vi "Main.vi"() -> ()   [LabVIEW 2020]
doc: "This template is for the Queued Message Handler design pattern.\n\nThe Event Handling Loop generates messages based on user interface actions.\n\nThe Message Handling Loop processes messages generated by the Event Handling Loop, or by other messages. The messages are string values, so new messages can be added easily to the Message Cases case structure in the Message Handling Loop. Each message cluster can also provide an optional value for Message Data, which is a variant that can be converted to whatever message-specific data is required."
uses:
  <vilib>/numeric/Random Number (Range) I64.vi
  <vilib>/numeric/sub_Random U32.vi
  <vilib>/Utility/error.llb/Error Cluster From Error Code.vi
  <vilib>/ErrorRing/Error Ring.xnode
  support/Message Queue/Message Queue.lvlib
  support/User Event - Stop/User Event - Stop.lvlib
panel:
  out "Order Array Display":string[](array[string])
  out "Button Array":refnum<vi>[](array[refnum])
  out "Stage Num":i32
  out "Click Num":i32
  out "Display <Replace Me>":string
  in  "Blue":bool
  in  "Red":bool
  in  "Exit":bool
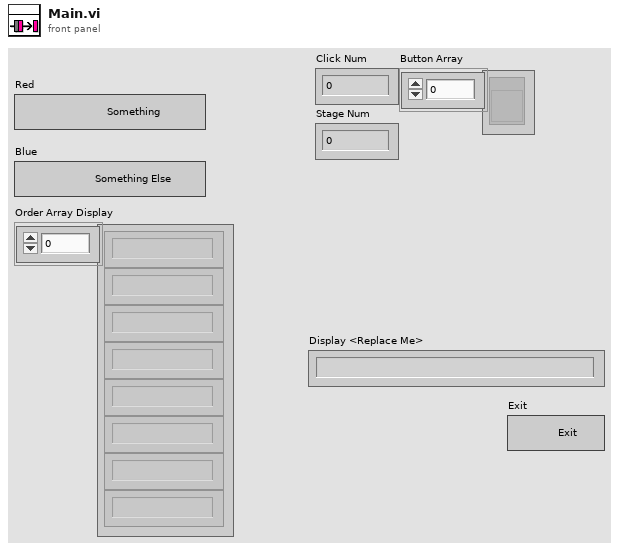
[diagram p1: front panel]
types:
  T1 = typedef "Message Queue.lvlib/All Message Queues.ctl" = cluster{"UI":refnum<queue>}
  T2 = enum8{"Enabled", "Disabled", "Disabled and Grayed Out"}
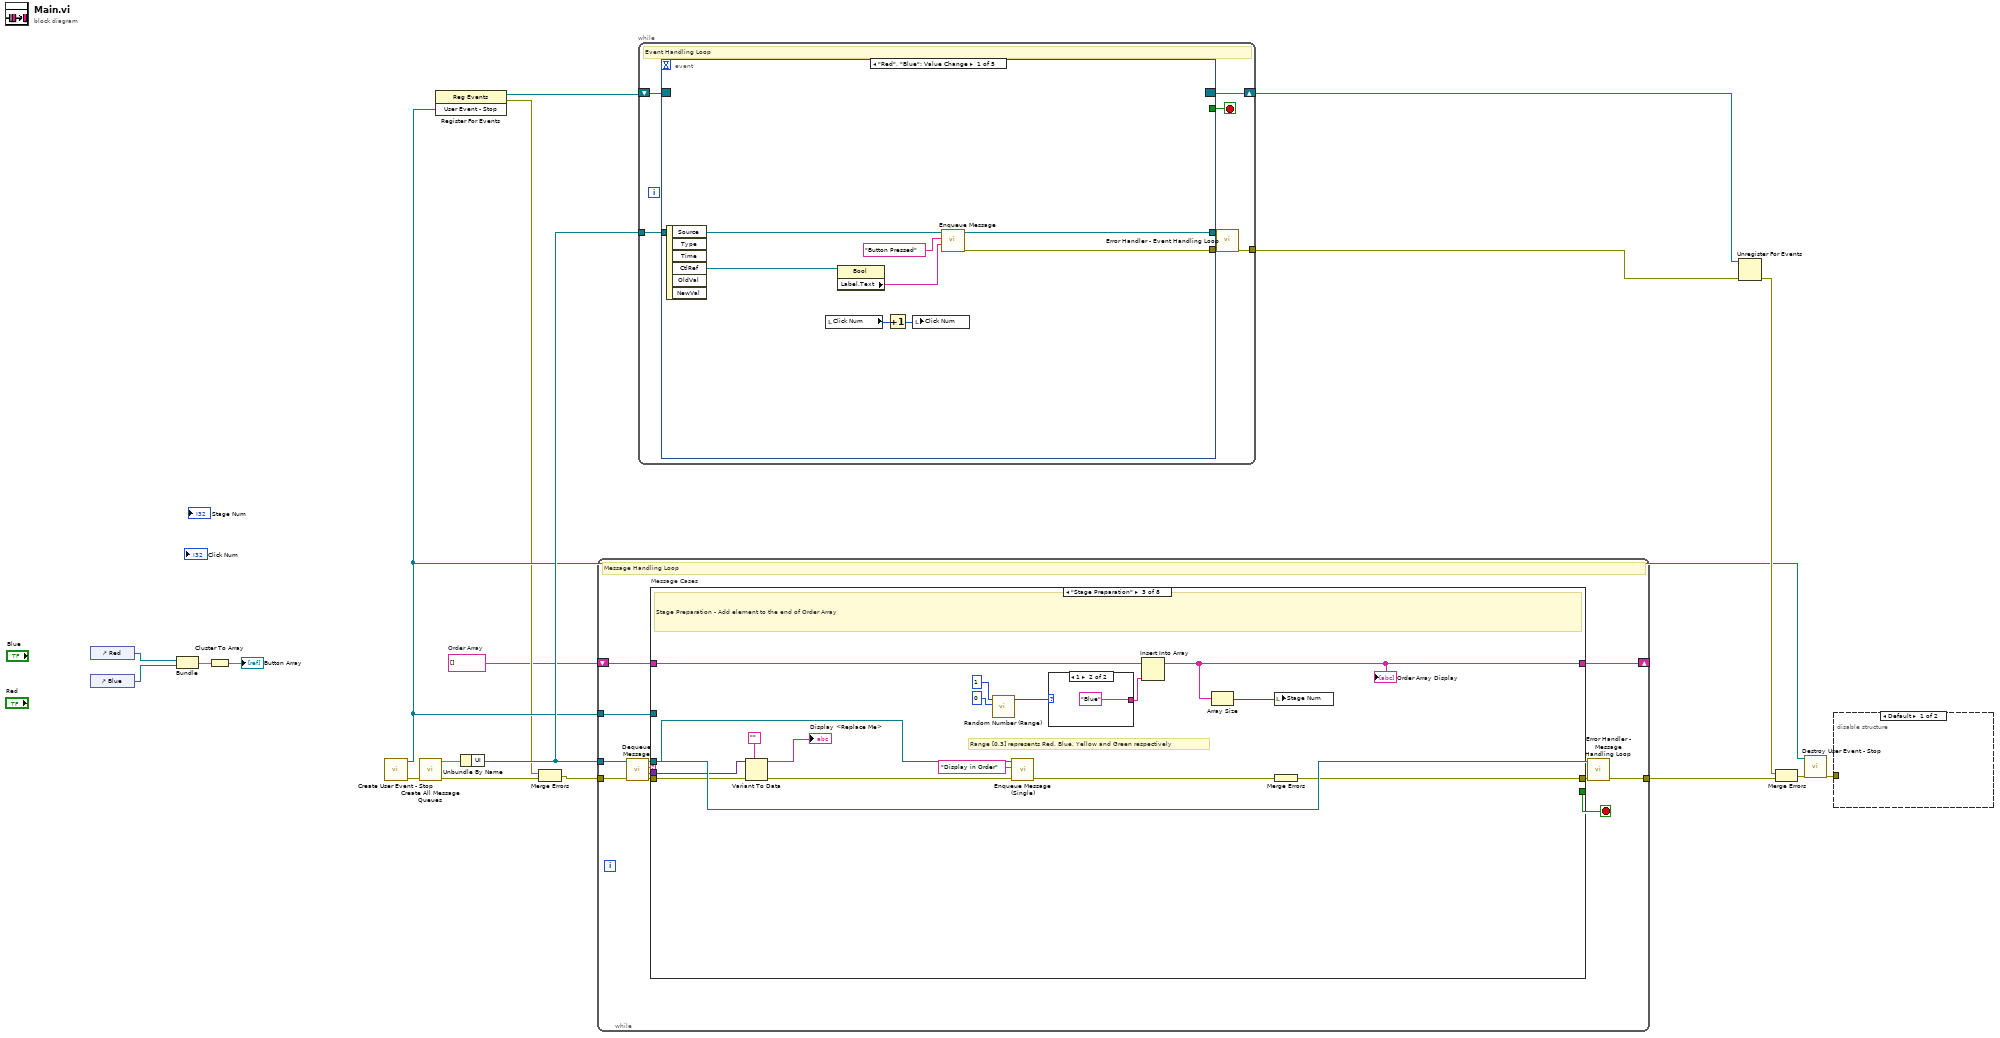
[diagram p0: block diagram]
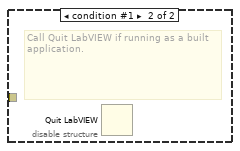
[diagram p2: hidden frame]
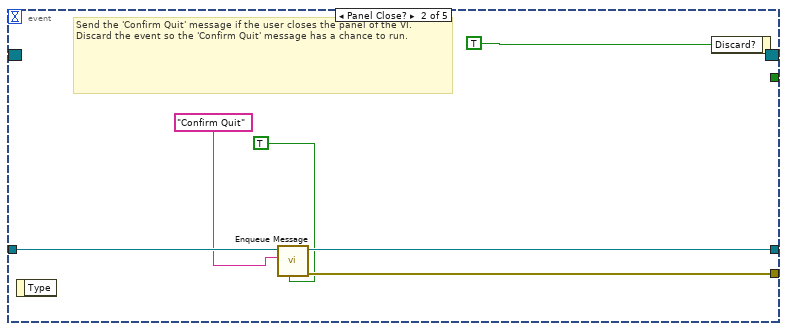
[diagram p3: hidden frame]
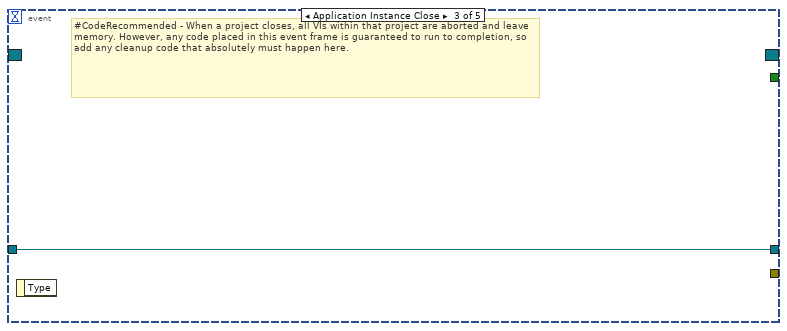
[diagram p4: hidden frame]
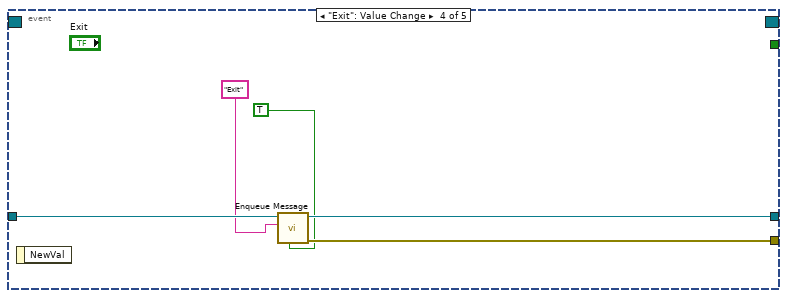
[diagram p5: hidden frame]
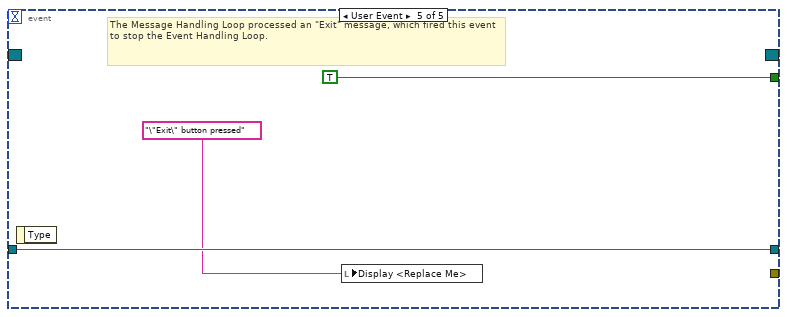
[diagram p6: hidden frame]
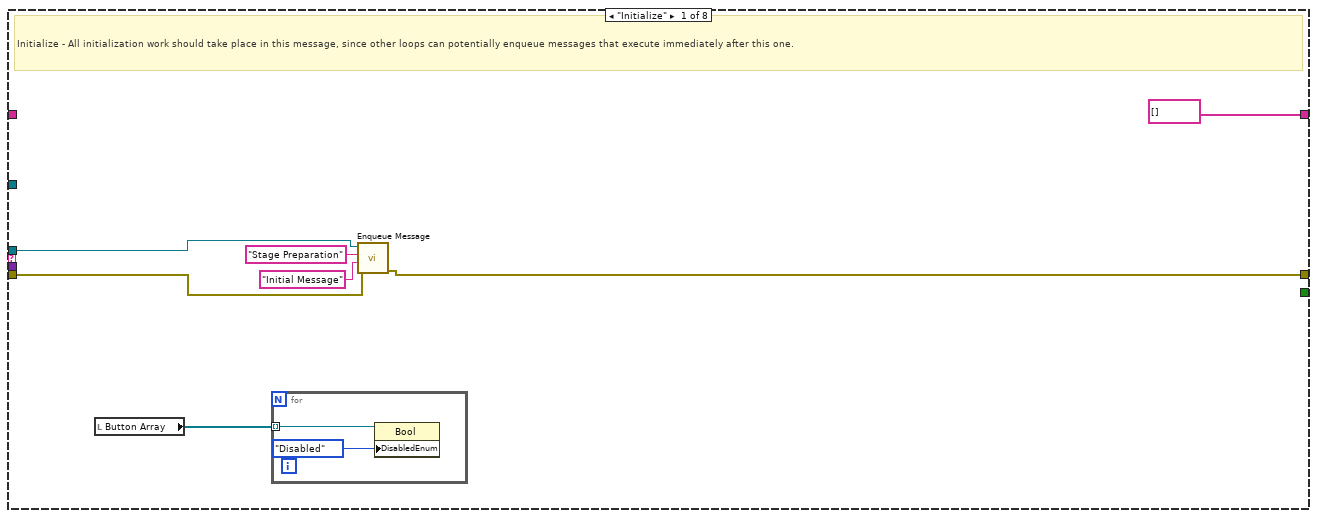
[diagram p7: hidden frame]
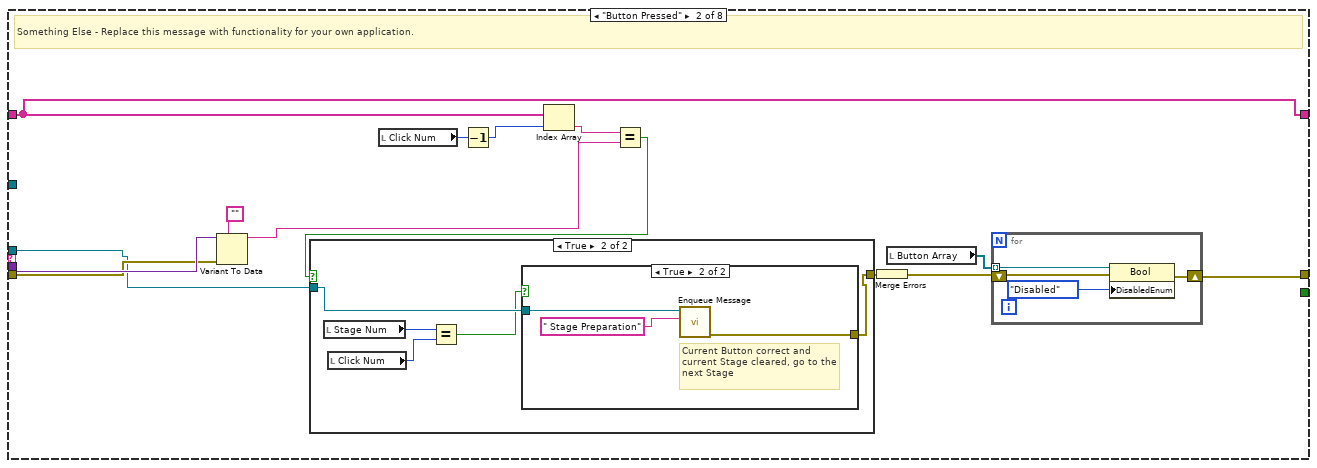
[diagram p8: hidden frame]
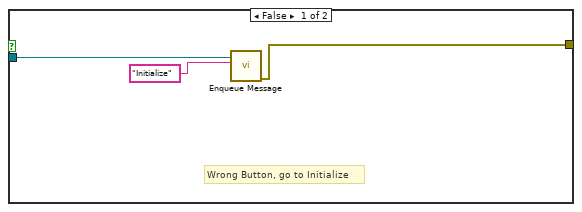
[diagram p9: hidden frame]
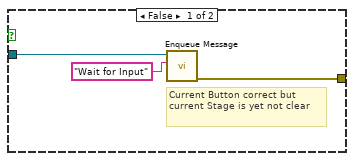
[diagram p10: hidden frame]
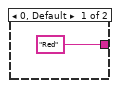
[diagram p11: hidden frame]
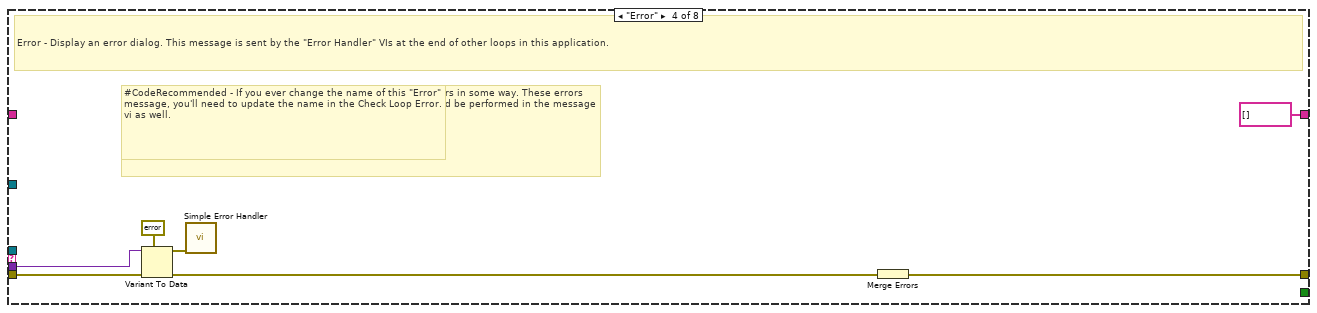
[diagram p12: hidden frame]
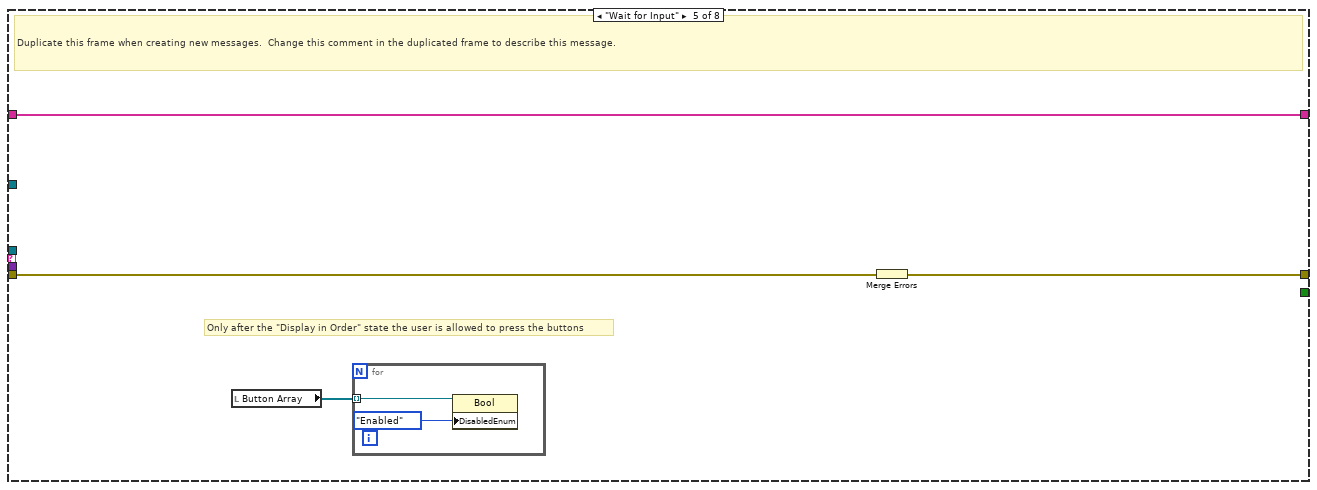
[diagram p13: hidden frame]
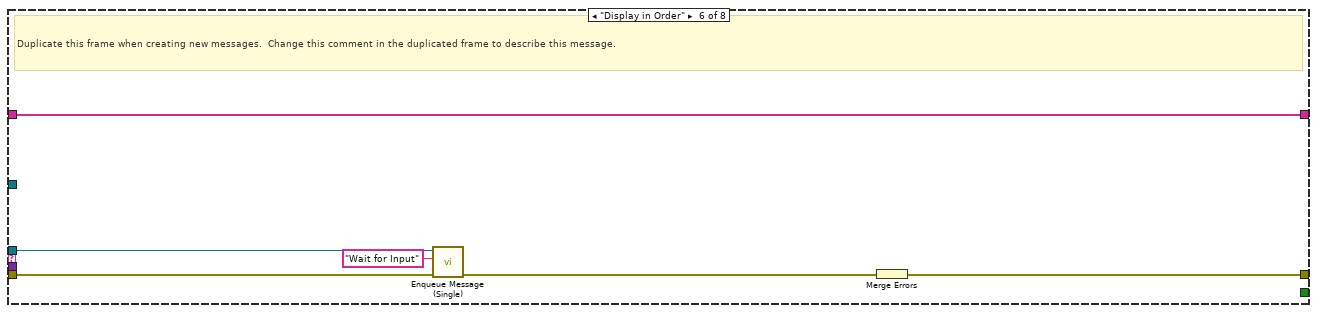
[diagram p14: hidden frame]
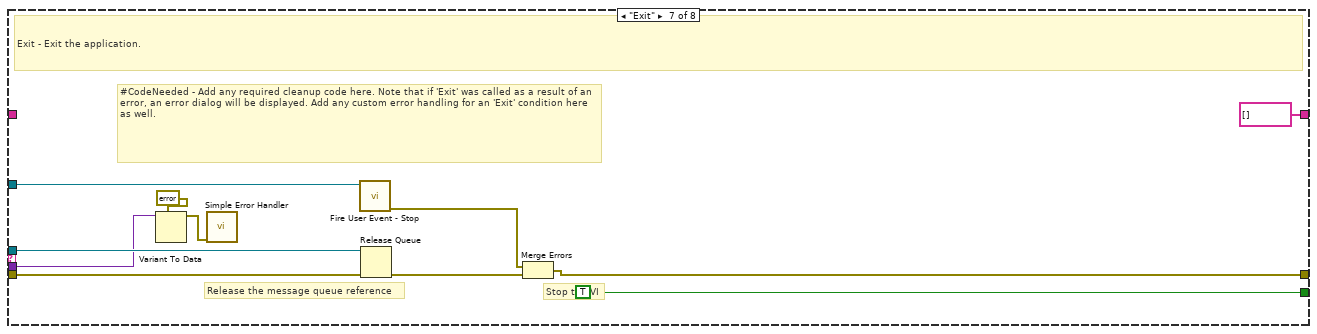
[diagram p15: hidden frame]
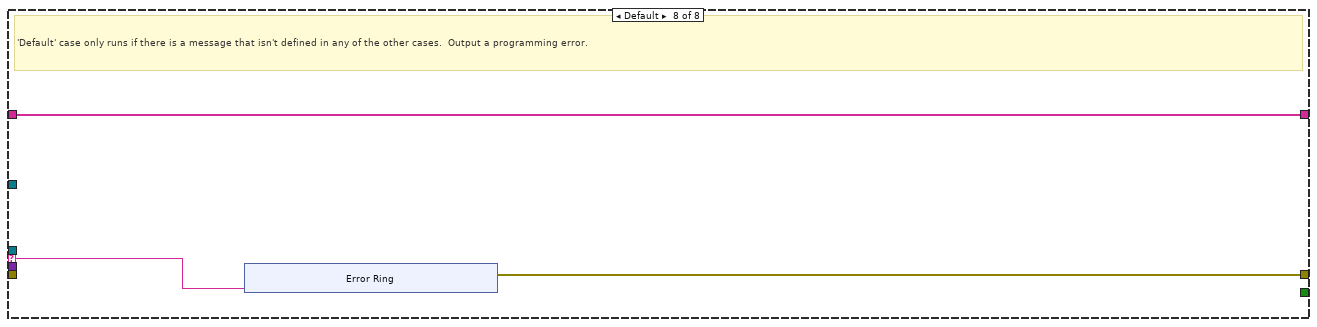
[diagram p16: hidden frame]
diagram:
  w5 = string[] []  # Order Array
  n1 = control-ref of="Red"() -> (w4:refnum<vi>)
  n2 = control-ref of="Blue"() -> (w3:refnum<vi>)
  n3 = Bundle("Red"=w4, "Blue"=w3) -> (w2:cluster{"Red":refnum<vi>, "Blue":refnum<vi>})  [unwired: 1 in]
  n4 = Cluster To Array(cluster=w2) -> (array=→"Button Array":refnum<vi>[])
  n5 = call "Create User Event - Stop.vi"() -> ("error out"=w15:errorcluster, "User Event - Stop"=w8:refnum<user-event>)  [unwired: 10 in]
  n6 = call "Create All Message Queues.vi"("error in (no error)"=w15) -> ("error out"=w19:errorcluster, "Message Queues out"=w18:T1)  [unwired: 9 in]
  n7 = register-events(w8) -> (reference out=w9:refnum<event-registration>, error out=w6:errorcluster)  [unwired: 2 in]
  n8 = Unbundle By Name(w18) -> ("UI"=w16:refnum<queue>)
  n9 = Merge Errors(w6, w19) -> (w7:errorcluster)
  n10 = while {
    tunnel: w16 -> [w25]
    tunnel: w8 -> [w30]
    tunnel: w7 -> [w29]
    tunnel: [w23] -> w17
    shift-right: [w20] -> _
    shift-left: w5 -> [w21]
    stop <- w31 stop-if-true
    # "Message Handling Loop"
    n11 = call "Dequeue Message.vi"("error in (no error)"=w29, "Message Queue"=w25) -> ("error out"=w28:errorcluster, "Message Data"=w26:variant, "Message"=w27:string, "dup Message Queue"=w24:refnum<queue>)  [unwired: 6 in]
    n12 = case "Message Cases" shown="\"Stage Preparation\"" w27 {
      selector: w27 -> [_ _ _ _ _ _ _ w122]
      tunnel: w24 -> [w35 w48 w74 _ _ w105 w120 _]
      tunnel: w28 -> [w37 w51 w87 w97 w101 w109 w114 _]
      tunnel: [w38 w42 w88 w92 w100 w108 w117 w123] -> w22
      tunnel: [_ _ _ _ _ _ TRUE _] -> w31
      tunnel: w26 -> [_ w52 w86 w96 _ _ w111 _]
      tunnel: w30 -> [_ _ _ _ _ _ w116 _]
      tunnel: w21 -> [_ w54 w82 _ w98 w107 _ w121]
      tunnel: [string[] [] w54 w77 string[] [] ("Order Array") w98 w107 string[] [] ("Order Array") w121] -> w20
      frame "Initialize" {
        # "Initialize - All initialization work should take place in this message, since other loops can potentially enqueue messages that execute immediately after this one."
        n13 = local read "Button Array"() -> (w33:refnum<vi>[])
        n14 = for {
          tunnel: w33 -> [w40] mode=indexing
          n15 = property class="Bool"(reference=w40, "DisabledEnum"=T2."Disabled" ("Disabled")) -> ()  [unwired: 1 in, 2 out]
        }
        n16 = call-poly "Enqueue Message.vi"("error in (no error)"=w37, "Message Data"="Initial Message" ("Initial Message"), "Message"="Stage Preparation", "Message Queue"=w35) -> ("error out"=w38:errorcluster)  [unwired: 6 in, 1 out]
      }
      frame "Button Pressed" {
        # "Something Else - Replace this message with functionality for your own application."
        n17 = Variant To Data(error in=w51, type="", Variant=w52) -> (data=w50:string)  [unwired: 1 out]
        n18 = local read "Click Num"() -> (w46:i32)
        n19 = Decrement(x=w46) -> (x-1=w45:i32)
        n20 = Index Array(array=w54, index=w45) -> (element=w44:string)
        n21 = Equal?(x=w44, y=w50) -> (x = y?=w49:bool)
        n22 = case shown="True" w49 {
          tunnel: w48 -> [w61 w65]
          tunnel: [w60 w66] -> w47
          frame False {
            # "Wrong Button, go to Initialize"
            n23 = call-poly "Enqueue Message.vi"("Message"="Initialize", "Message Queue"=w61) -> ("error out"=w60:errorcluster)  [unwired: 8 in, 1 out]
          }
          frame True {
            n24 = local read "Stage Num"() -> (w64:i32)
            n25 = local read "Click Num"() -> (w63:i32)
            n26 = Equal?(x=w64, y=w63) -> (x = y?=w62:bool)
            n27 = case shown="True" w62 {
              tunnel: [w69 w71] -> w66
              tunnel: w65 -> [w67 w72]
              frame False {
                # "Current Button correct but \ncurrent Stage is yet not clear"
                n28 = call-poly "Enqueue Message.vi"("Message"="Wait for Input", "Message Queue"=w67) -> ("error out"=w69:errorcluster)  [unwired: 8 in, 1 out]
              }
              frame True {
                # "Current Button correct and \ncurrent Stage cleared, go to the next Stage"
                n29 = call-poly "Enqueue Message.vi"("Message"=" Stage Preparation", "Message Queue"=w72) -> ("error out"=w71:errorcluster)  [unwired: 8 in, 1 out]
              }
            }
          }
        }
        n30 = Merge Errors(w47) -> (w43:errorcluster)
        n31 = local read "Button Array"() -> (w41:refnum<vi>[])
        n32 = for {
          tunnel: w41 -> [w58] mode=indexing
          shift-right: [w55] -> w42
          shift-left: w43 -> [w56]
          n33 = property class="Bool"(reference=w58, error in=w56, "DisabledEnum"=T2."Disabled" ("Disabled")) -> (error out=w55:errorcluster)  [unwired: 1 out]
        }
      }
      frame "Stage Preparation" {
        # "Range [0,3] represents Red, Blue, Yellow and Green respectively"
        # "Stage Preparation - Add element to the end of Order Array"
        n34 = Variant To Data(error in=w87, type="", Variant=w86) -> (data=→"Display <Replace Me>":string, error out=w84:errorcluster)
        n35 = call-poly <vilib>:"Random Number (Range).vi"("lower bound (-100)"=i64 0, "upper bound (100)"=i64 1) -> ("number"=w79:i64)  [unwired: 9 in]
        n36 = call "Enqueue Message (Single).vi"("error in (no error)"=w84, "Message"="Display in Order", "Message Queue"=w74) -> ("error out"=w75:errorcluster)  [unwired: 7 in, 1 out]
        n37 = case shown="1" w79 {
          tunnel: ["Red" "Blue"] -> w78
          frame 0, Default {
          }
          frame 1 {
          }
        }
        n38 = Insert Into Array(array=w82, new element=w78) -> (w77:string[])  [unwired: 1 in]
        "Order Array Display" <- w77
        n39 = Array Size(array=w77) -> (size(s)=w76:i32)
        n40 = local write "Stage Num"(w76) -> ()
        n41 = Merge Errors(w75) -> (w88:errorcluster)
      }
      frame "Error" {
        # "#CodeRecommended - If you ever change the name of this \"Error\" message, you'll need to update the name in the Check Loop Error.vi as well."
        # "#CodeRecommended - Consider creating a system for logging errors in some way. These errors are for notification purposes only. Handling of specific errors should be performed in the message frames that generated the error."
        # "Error - Display an error dialog. This message is sent by the \"Error Handler\" VIs at the end of other loops in this application."
        n42 = Variant To Data(error in=w97, type=errorcluster {"status"=FALSE, "code"=0, "source"=""} ("error constant"), Variant=w96) -> (data=w94:errorcluster, error out=w93:errorcluster)
        n43 = call <vilib>:"Simple Error Handler.vi"("error in (no error)"=w94) -> ()  [unwired: 4 in, 5 out]
        n44 = Merge Errors(w93) -> (w92:errorcluster)
      }
      frame "Wait for Input" {
        # "Only after the \"Display in Order\" state the user is allowed to press the buttons"
        # "Duplicate this frame when creating new messages.  Change this comment in the duplicated frame to describe this message."
        n45 = local read "Button Array"() -> (w99:refnum<vi>[])
        n46 = for {
          tunnel: w99 -> [w103] mode=indexing
          n47 = property class="Bool"(reference=w103, "DisabledEnum"=T2."Enabled" ("Disabled")) -> ()  [unwired: 1 in, 2 out]
        }
        n48 = Merge Errors(w101) -> (w100:errorcluster)
      }
      frame "Display in Order" {
        # "Duplicate this frame when creating new messages.  Change this comment in the duplicated frame to describe this message."
        n49 = call "Enqueue Message (Single).vi"("error in (no error)"=w109, "Message"="Wait for Input", "Message Queue"=w105) -> ("error out"=w106:errorcluster)  [unwired: 7 in, 1 out]
        n50 = Merge Errors(w106) -> (w108:errorcluster)
      }
      frame "Exit" {
        # "Stop the VI"
        # "Release the message queue reference"
        # "#CodeNeeded - Add any required cleanup code here. Note that if 'Exit' was called as a result of an error, an error dialog will be displayed. Add any custom error handling for an 'Exit' condition here as well."
        # "Exit - Exit the application."
        n51 = Variant To Data(type=errorcluster {"status"=FALSE, "code"=0, "source"=""} ("error constant"), Variant=w111) -> (data=w112:errorcluster)  [unwired: 1 in, 1 out]
        n52 = call <vilib>:"Simple Error Handler.vi"("error in (no error)"=w112) -> ()  [unwired: 4 in, 5 out]
        n53 = call "Fire User Event - Stop.vi"("User Event - Stop"=w116) -> ("error out"=w115:errorcluster)  [unwired: 10 in]
        n54 = Release Queue(queue=w120, error in (no error)=w114) -> (error out=w118:errorcluster)  [unwired: 1 in, 2 out]
        n55 = Merge Errors(w115, w118) -> (w117:errorcluster)
      }
      frame Default {
        # "'Default' case only runs if there is a message that isn't defined in any of the other cases.  Output a programming error."
        n56 = xnode "Error Ring"("parameter 0"=w122) -> ("error out"=w123:errorcluster)
      }
    }
    n57 = call "Error Handler - Message Handling Loop.vi"("error in (no error)"=w22, "Message Queue"=w24) -> ("dup error in"=w23:errorcluster)  [unwired: 8 in, 1 out]
  }
  n58 = while {
    tunnel: w16 -> [w137]
    shift-right: [w135] -> w12
    shift-left: w9 -> [w136]
    tunnel: [w131] -> w10
    stop <- w133 stop-if-true
    # "Event Handling Loop"
    n59 = event shown="[0] \"Red\", \"Blue\": Value Change" {
      selector: w136 -> [_ _ _ _ _]
      dyn-events: [_ _ _ _ _] -> w135
      timeout: _ -> [_ _ _ _ _]
      tunnel: [_ _ _ _ TRUE ("Discard?")] -> w133
      tunnel: w137 -> [w145 w150 w152 w157 w160]
      tunnel: [w143 w149 _ w156 _] -> w134
      tunnel: [w144 w148 w152 w155 w160] -> w132
      event "Red", "Blue": Value Change {
        n60 = event-data() -> ("CtlRef"=w142:refnum<vi>)  [unwired: 1 in, 5 out]
        n61 = local read "Click Num"() -> (w138:i32)
        n62 = property class="Bool"(reference=w142) -> ("Label.Text"=w140:string)  [unwired: 1 in, 2 out]
        n63 = Increment(x=w138) -> (x+1=w139:i32)
        n64 = local write "Click Num"(w139) -> ()
        n65 = call-poly "Enqueue Message.vi"("Message Data"=w140, "Message"="Button Pressed", "Message Queue"=w145) -> ("error out"=w143:errorcluster, "dup Message Queue"=w144:refnum<queue>)  [unwired: 7 in]
      }
      event Panel Close? {
        # "Send the 'Confirm Quit' message if the user closes the panel of the VI. Discard the event so the 'Confirm Quit' message has a chance to run."
        n66 = event-data() -> ()  [unwired: 1 in, 1 out]
        n67 = call-poly "Enqueue Message.vi"("Priority Message? (F)"=TRUE, "Message"="Confirm Quit", "Message Queue"=w150) -> ("error out"=w149:errorcluster, "dup Message Queue"=w148:refnum<queue>)  [unwired: 7 in]
        n68 = event-data("Discard?"=TRUE) -> ()  [unwired: 1 in, 1 out]
      }
      event Application Instance Close {
        # "#CodeRecommended - When a project closes, all VIs within that project are aborted and leave memory. However, any code placed in this event frame is guaranteed to run to completion, so add any cleanup code that absolutely must happen here."
        n69 = event-data() -> ()  [unwired: 1 in, 1 out]
      }
      event "Exit": Value Change {
        n70 = event-data() -> ()  [unwired: 1 in, 1 out]
        n71 = call-poly "Enqueue Message.vi"("Priority Message? (F)"=TRUE, "Message"="Exit", "Message Queue"=w157) -> ("error out"=w156:errorcluster, "dup Message Queue"=w155:refnum<queue>)  [unwired: 7 in]
      }
      event User Event {
        # "The Message Handling Loop processed an \"Exit\" message, which fired this event to stop the Event Handling Loop."
        n72 = event-data() -> ()  [unwired: 1 in, 1 out]
        n73 = local write "Display <Replace Me>"("\"Exit\" button pressed" ("VI Stopped")) -> ()
      }
    }
    n74 = call "Error Handler - Event Handling Loop.vi"("error in (no error)"=w134, "Message Queue"=w132) -> ("dup error in"=w131:errorcluster)  [unwired: 8 in, 1 out]
  }
  n75 = Unregister For Events(event registration refnum=w12, error in=w10) -> (error out=w13:errorcluster)
  n76 = Merge Errors(w13, w17) -> (w14:errorcluster)
  n77 = call "Destroy User Event - Stop.vi"("error in (no error)"=w14, "User Event - Stop"=w8) -> ("error out"=w11:errorcluster)  [unwired: 9 in]
  n78 = disable-structure shown="Default" {
    disable-tunnel: w11 -> [_ _]
    frame condition #0 (active) {
    }
    frame condition #1 {
      # "Call Quit LabVIEW if running as a built application."
      n79 = Quit LabVIEW() -> ()  [unwired: 1 in]
    }
  }
